vi "Write Test Status.vi"(8 "error in (no error)":errorcluster, 11 "Model in":refnum<class "Model.lvclass">) -> (0 "error out":errorcluster, 3 "Model out":refnum<class "Model.lvclass">)   [LabVIEW 2016, in "Model.lvclass"]
uses:
  Model.lvclass
  Model.lvclass/Model.ctl
  Test Log/Test Log/Test Log.lvclass
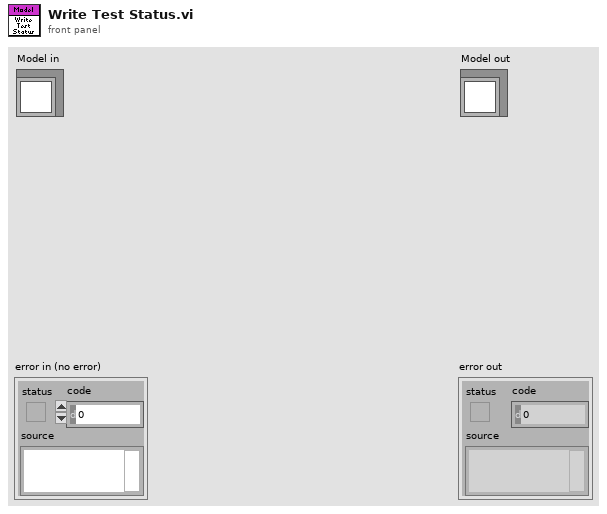
[diagram p1: front panel]
types:
  T1 = typedef "HPMT_Typedefs.lvlib/TestStatus.ctl" = enum16{"Not Run", "Running", "Passed", "Failed"}
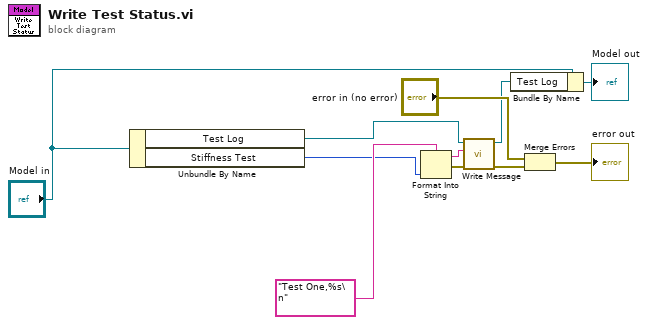
[diagram p0: block diagram]
diagram:
  n1 = Unbundle By Name("Model in") -> ("Test Log"=w3:refnum<class "Test Log.lvclass">, "Stiffness Test"=w8:T1)
  n2 = Format Into String(format string="Test One,%s\n", w8) -> (resulting string=w7:string, error out=w6:errorcluster)  [unwired: 2 in]
  n3 = call-dynamic "Write Message.vi"("error in (no error)"=w6, "Message"=w7, "Test Log in"=w3) -> ("error out"=w5:errorcluster, "Test Log out"=w2:refnum<class "Test Log.lvclass">)  [unwired: 7 in]
  n4 = Bundle By Name(cluster="Model in", "Test Log"=w2) -> (→"Model out":refnum<class "Model.lvclass">)
  n5 = Merge Errors("error in (no error)", w5) -> (→"error out":errorcluster)
